vi "2 SiO2 Material Properties.vi"(6 "NS Base Area":dbl, 9 "m-nm SiO2 in":dbl, 10 "Silicon DiOxide Thickness  in":dbl, 11 "Energy (Heat; I^2R)":dbl) -> (1 "Volume SiO2 2":dbl, 2 "SiO2 Specfic Heat Capacity 2":dbl, 3 "Mass SiO2 2":dbl, 4 "SiO2 Thickness 2":dbl, 5 "Delta Temp Change SiO2 2":dbl, 7 "SilO2 Density 2":dbl)   [LabVIEW 2020]
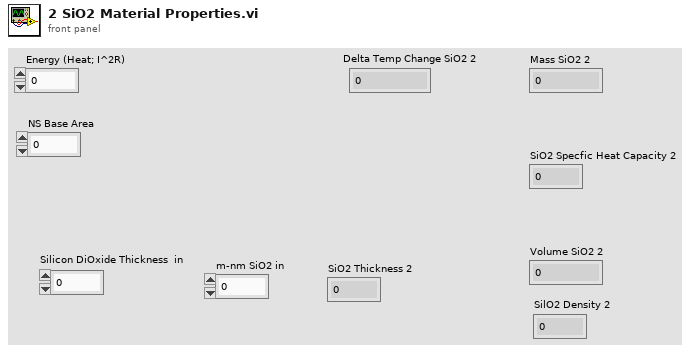
[diagram p1: front panel]
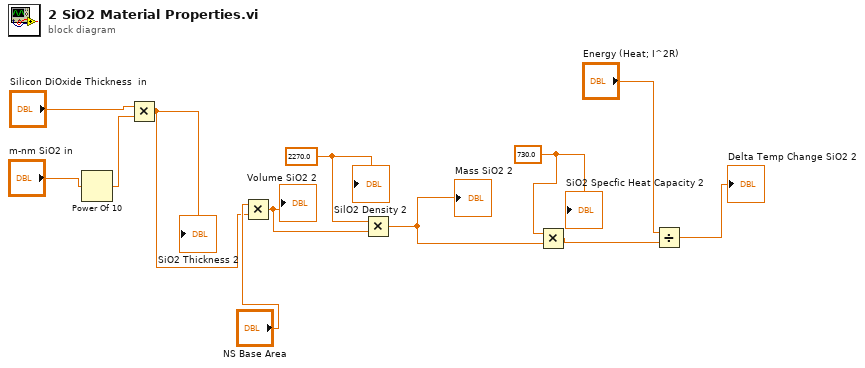
[diagram p0: block diagram]
diagram:
  w6 = 730.0 ("Silicon Specfic Heat Capacity 2")
  w4 = 2270.0 ("Silicon Dioxide Density 2")
  n1 = Power Of 10(x="m-nm SiO2 in") -> (10^x=w1:dbl)
  n2 = Multiply(x="Silicon DiOxide Thickness  in", y=w1) -> (x*y=w10:dbl)
  "SiO2 Thickness 2" <- w10
  n3 = Multiply(x="NS Base Area", y=w10) -> (x*y=w5:dbl)
  "Volume SiO2 2" <- w5
  n4 = Multiply(x=w4, y=w5) -> (x*y=w9:dbl)
  "Mass SiO2 2" <- w9
  n5 = Multiply(x=w6, y=w9) -> (x*y=w8:dbl)
  n6 = Divide(x="Energy (Heat; I^2R)", y=w8) -> (x/y=→"Delta Temp Change SiO2 2":dbl)
  "SilO2 Density 2" <- w4
  "SiO2 Specfic Heat Capacity 2" <- w6
